vi "Close.vi"(8 "error in (no error)":errorcluster, 11 "LabVEIW Instance in":refnum<class "LabVIEW Instance.lvclass">) -> (0 "error out":errorcluster)   [LabVIEW 2014, in "LabVIEW Instance.lvclass"]
uses:
  LabVIEW Instance.lvclass
  LabVIEW Instance.lvclass/LabVIEW Instance.ctl
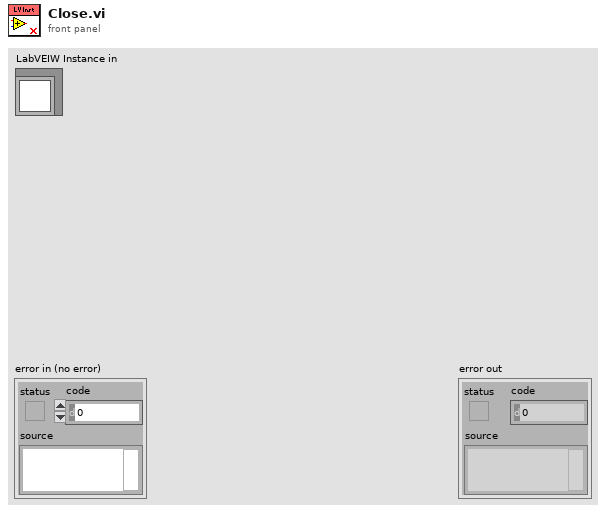
[diagram p1: front panel]
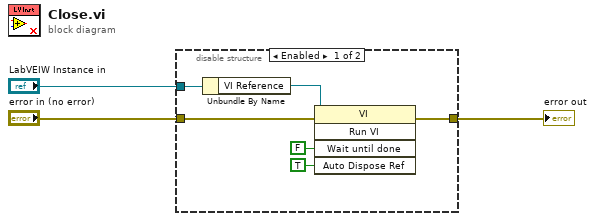
[diagram p0: block diagram]
diagram:
  n1 = disable-structure shown="Enabled" {
    disable-tunnel: "error in (no error)" -> [w9 _]
    disable-tunnel: [w8 _] -> w2
    disable-tunnel: "LabVEIW Instance in" -> [w7 _]
    frame Enabled {
      n2 = Unbundle By Name(w7) -> ("VI Reference"=w6:refnum<vi>)
      n3 = invoke class="VI" method="Run VI"(reference=w6, error in=w9, "Wait until done"=FALSE ("Wait Until Done"), "Auto Dispose Ref"=TRUE ("Auto Dispose Reference")) -> (error out=w8:errorcluster)  [unwired: 1 in, 4 out]
    }
    frame Disabled {
    }
  }
  "error out" <- w2
